vi "IScanStop.vi"(0 "PRIORLib.IScanIn":refnum<k7>) -> (1 "PRIORLib.IScanOut":refnum<k7>, 2 "error out":errorcluster, 3 "Return":i32)   [LabVIEW 2011]
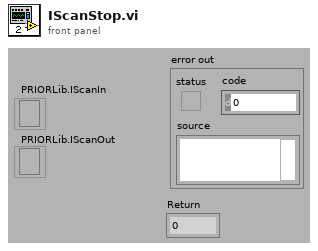
[diagram p1: front panel]
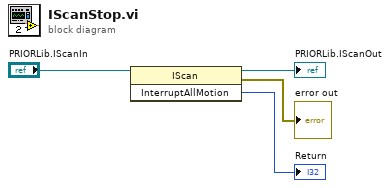
[diagram p0: block diagram]
diagram:
  n1 = invoke class="IScan" method="InterruptAllMotion"(reference="PRIORLib.IScanIn") -> (reference out=→"PRIORLib.IScanOut":refnum<k7>, error out=→"error out":errorcluster, "InterruptAllMotion"=→"Return":i32)  [unwired: 2 in]
